vi "Quadratic_eq.vi"() -> ()   [LabVIEW 2026]
panel:
  out "String":string
  out "Root 2":dbl
  out "Root 1":dbl
  in  "c":dbl
  in  "b":dbl
  in  "a":dbl
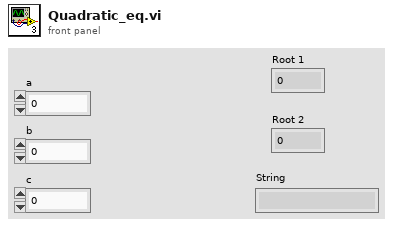
[diagram p1: front panel]
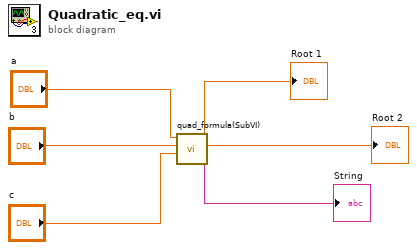
[diagram p0: block diagram]
diagram:
  n1 = call "quad_formula(SubVI).vi"("c"="c", "b"="b", "a"="a") -> ("String"=→"String":string, "Numeric"=→"Root 2":dbl, "Numeric 2"=→"Root 1":dbl)  [unwired: 6 in]
